vi "主副屏通信slave.vi"() -> ()   [LabVIEW 2016, in "斯坦道多参数.lvlib"]
uses:
  <vilib>/NI/Modbus Library/API/Wrapper/Create TCP Slave.vi
  <vilib>/NI/Modbus Library/API/slave/Modbus Slave.lvclass
  <vilib>/NI/Modbus Library/API/Wrapper/API Main.lvlib
panel:
  in  "停止":bool
  out "read values":u16[](array[numeric])
  in  "write values":u16[](array[numeric])
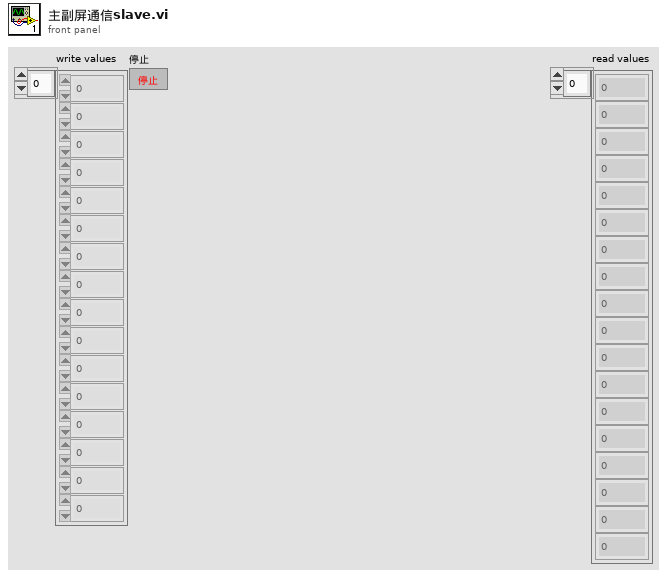
[diagram p1: front panel]
types:
  T1 = cluster{"数据保存间隔":dbl, "水温标样值":dbl, "pH标样值":dbl, "溶解氧标样值":dbl, "电导率标样值":dbl, "浊度标样值":dbl}
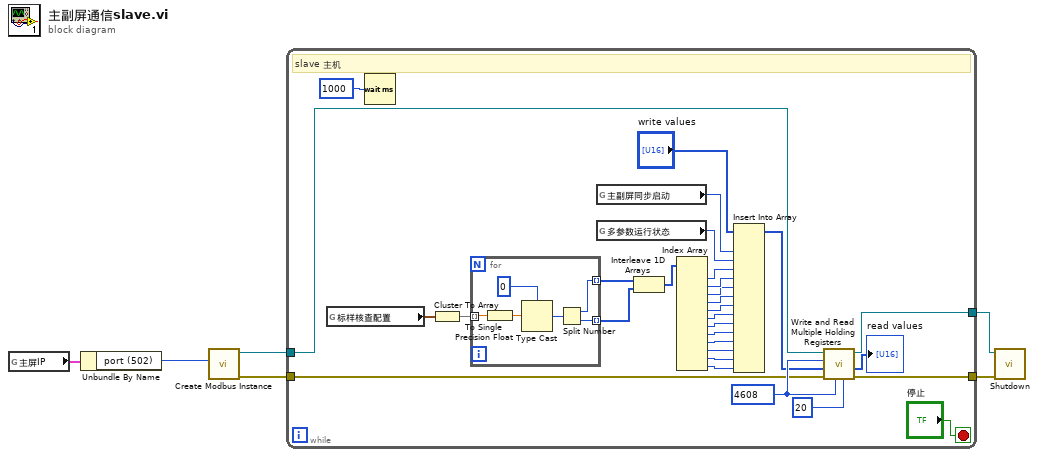
[diagram p0: block diagram]
diagram:
  n1 = global read "多参数全局变量.vi" "主屏IP"() -> (w2:cluster{"address":string, "port (502)":u16})
  n2 = Unbundle By Name(w2) -> ("port (502)"=w1:u16)
  n3 = call-poly <vilib>:"Create Modbus Instance.vi"("port (502)"=w1) -> ("error out"=w3:errorcluster, "TCP slave instance"=w6:refnum<class "Modbus Slave.lvclass">)  [unwired: 9 in]
  n4 = while {
    tunnel: w6 -> [w28]
    tunnel: [w33] -> w5
    tunnel: [w32] -> w4
    tunnel: w3 -> [w31]
    stop <- "停止" stop-if-true
    w36 = u16 4608 ("write starting address")
    # "slave 主机"
    n5 = global read "断电保存变量.vi" "标样核查配置"() -> (w23:T1)
    n6 = Wait (ms)(milliseconds to wait=u32 1000 ("等待时间（毫秒）")) -> ()  [unwired: 1 out]
    n7 = Cluster To Array(cluster=w23) -> (array=w22:dbl[])
    n8 = for {
      tunnel: w22 -> [w38] mode=indexing
      tunnel: [w40] -> w21 mode=indexing
      tunnel: [w39] -> w20 mode=indexing
      n9 = To Single Precision Float(number=w38) -> (single precision float=w37:sgl)
      n10 = Type Cast(type=0, x=w37) -> (*(type *) &x=w41:i32)
      n11 = Split Number(x=w41) -> (hi(x)=w40:u16, lo(x)=w39:u16)
    }
    n12 = global read "多参数全局变量.vi" "主副屏同步启动"() -> (w25:u16)
    n13 = global read "多参数全局变量.vi" "多参数运行状态"() -> (w24:u16)
    n14 = Interleave 1D Arrays(w21, w20) -> (w19:u16[])
    n15 = Index Array(array=w19) -> (element #1=w18:u16, element #2=w17:u16, element #3=w16:u16, element #4=w15:u16, element #5=w14:u16, element #6=w13:u16, element #7=w12:u16, element #8=w11:u16, element #9=w10:u16, element #10=w9:u16, element #11=w8:u16, element #12=w7:u16)  [unwired: 12 in]
    n16 = Insert Into Array(array="write values", new element #1=w25, new element #2=w24, new element #3=w18, new element #4=w17, new element #5=w16, new element #6=w15, new element #7=w14, new element #8=w13, new element #9=w12, new element #10=w11, new element #11=w10, new element #12=w9, new element #13=w8, new element #14=w7) -> (w26:u16[])  [unwired: 1 in]
    n17 = call-dynamic "Write and Read Multiple Holding Registers.vi"("read count"=u16 20, "read starting address"=w36, "error in"=w31, "write values"=w26, "write starting address"=w36, "Modbus instance in"=w28) -> ("error out"=w32:errorcluster, "read values"=→"read values":u16[], "Modbus instance out"=w33:refnum<class "Modbus Slave.lvclass">)  [unwired: 3 in]
  }
  n18 = call-dynamic "Shutdown.vi"("error in"=w4, "Modbus slave in"=w5) -> ()  [unwired: 9 in, 1 out]
